vi "CarFrontPanel.vi"() -> ()   [LabVIEW 2017]
panel:
  out "Boolean":bool
  in  "Down":bool
  in  "Up":bool
  out "Marcia":dbl
  out "Numero di giri":dbl(knob) scale=0.0..300.0
  in  "stop":bool
  in  "Acceleratore":dbl(slide) scale=0.0..10.0
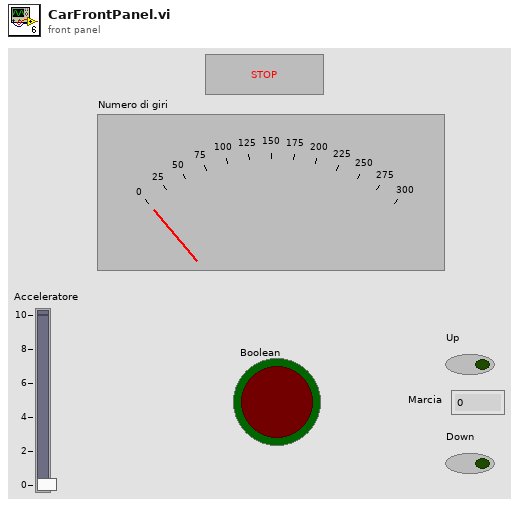
[diagram p1: front panel]
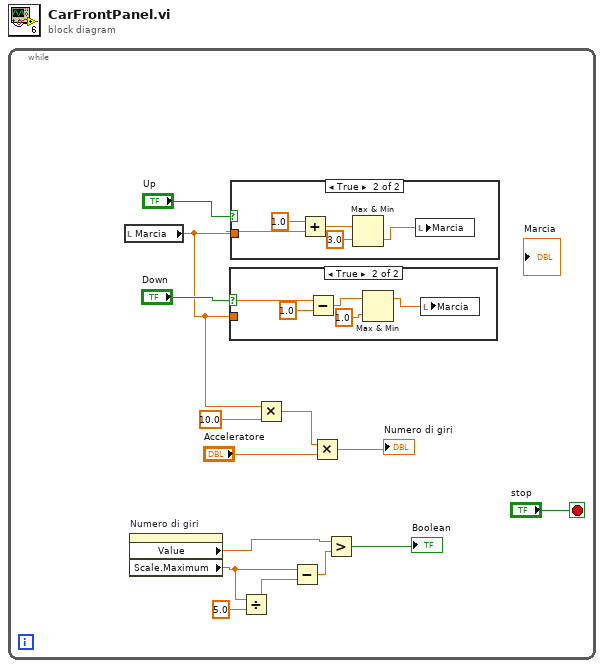
[diagram p0: block diagram]
diagram:
  n1 = while {
    stop <- "stop" stop-if-true
    n2 = local read "Marcia"() -> (w11:dbl)
    n3 = property on="Numero di giri" class="Knob (strict)"() -> ("Value"=w6:dbl, "Scale.Maximum"=w4:dbl)  [unwired: 2 in, 2 out]
    n4 = case shown="True" "Down" {
      tunnel: w11 -> [_ w19]
      frame False {
      }
      frame True {
        n5 = Subtract(x=w19, y=1.0) -> (x-y=w17:dbl)
        n6 = Max & Min(x=w17, y=1.0) -> (max(x,y)=w15:dbl)  [unwired: 1 out]
        n7 = local write "Marcia"(w15) -> ()
      }
    }
    n8 = case shown="True" "Up" {
      tunnel: w11 -> [_ w24]
      frame False {
      }
      frame True {
        n9 = Add(x=1.0, y=w24) -> (x+y=w22:dbl)
        n10 = Max & Min(x=w22, y=3.0) -> (min(x,y)=w20:dbl)  [unwired: 1 out]
        n11 = local write "Marcia"(w20) -> ()
      }
    }
    n12 = Divide(x=w4, y=5.0) -> (x/y=w2:dbl)
    n13 = Multiply(x=w11, y=10.0) -> (x*y=w9:dbl)
    n14 = Subtract(x=w4, y=w2) -> (x-y=w1:dbl)
    n15 = Multiply(x=w9, y="Acceleratore") -> (x*y=→"Numero di giri":dbl)
    n16 = Greater?(x=w6, y=w1) -> (0:→"Boolean":bool)
  }
